vi "Append Paragraph.vi"(0 "PDF Report":refnum<class "PDF Report Class.lvclass">, 1 "Path":path, 2 "Text":string, 3 "Paragraph indentation":T3, 7 "Image to Add [ ]":T1 {"Scale" format="%#_g %"}, 11 "error in (no error)":errorcluster, 12 "Font":T7={"Name"="", "Size"=-1.0, "Color"=0, "Style"={"Bold"=FALSE, "Italic"=FALSE, "Underline"=FALSE, "Strikeout"=FALSE}, "Type"={"Type&direction"=enum."Select", "Embedded"=FALSE, "Encoding"=""}}, 14 "Paragraph properties":T4) -> (4 "PDF Report duplicate":refnum<class "PDF Report Class.lvclass">, 15 "error out":errorcluster)   [LabVIEW 2020, in "Exaprom PDF.lvlib"]
doc: "<B>Only ASCII or UTF-16 (no-bidi).</B>\n\nAppends text with a <B>line feed</B>, at the end, to the PDF report. This text can be <B>aligned</B> (CENTER, JUSTIFY, LEFT, RIGHT) and <B>indented</B>. \n\nIf <B>Font</B> and <B>Pararaph properties</B> are not specified then the <B>Default font</B> and <B>Default paragraph</B> will be use.\n\nThe data type you wire to the <B>Text</B> input determines the polymorphic instance to use.\n\n<B>FRANÇAIS</B>\nAjoute au rapport PDF du texte sous la forme d'un paragraphe terminé avec un \"<B>Line Feed</B>\". Ce texte peut être <B>aligné</B> (CENTER, JUSTIFY, LEFT, RIGHT) et avoir un <B>renfoncement</B> (gauche et droit) pour tout le paragraphe.\n\nSi la police de caractères <B>Font</B> et les propriétés <B>Pararaph properties</B> ne sont pas spécifiés alors la police par défaut <B>Default font</B> et <B>Default paragraph</B> seront utilisées.\n\nLe type de données que vous connectez au terminal <B>Text</B> détermine l'instance polymorphique utilisée.\n\nVersion 2.0\nDeveloped by Jean-Marc Simard\nCopyright © 2013, Exaprom Inc.\nAll rights reserved.\nLicense: BSD\n\nWith iTextSharp 4.1.6 (http://itextsharp.sourceforge.net)\nunder Mozilla Public License Version 1.1\n(http://www.mozilla.org/MPL/MPL-1.1.html)"
uses:
  <userlib>/labview-PDF-writer-master/Exaprom PDF.lvlib
  <userlib>/labview-PDF-writer-master/Controls/Font Controls/Font complete cluster.ctl
  <userlib>/labview-PDF-writer-master/Controls/Font Controls/Font size.ctl
  <userlib>/labview-PDF-writer-master/Controls/Font Controls/Font color.ctl
  <userlib>/labview-PDF-writer-master/Controls/Font Controls/Type and encoding.ctl
  <userlib>/labview-PDF-writer-master/Controls/Text Controls/Unicode/Type and run direction.ctl
  <userlib>/labview-PDF-writer-master/Controls/Initialization Controls/Defaut Paragraphe and Line Spacing.ctl
  <userlib>/labview-PDF-writer-master/Controls/Text Controls/Texte alignement.ctl
  <userlib>/labview-PDF-writer-master/Controls/Text Controls/Line spacing.ctl
  <userlib>/labview-PDF-writer-master/LV Class/PDF Report Class/PDF Report Class.lvclass
  <userlib>/labview-PDF-writer-master/Controls/Text Controls/Paragraph indentation.ctl
  <userlib>/labview-PDF-writer-master/Controls/General Controls/Image to Add [ ].ctl
  <userlib>/labview-PDF-writer-master/Controls/Image Controls/Image Scale.ctl
  <userlib>/labview-PDF-writer-master/Controls/Text Controls/Phrase or paragraph.ctl
  <userlib>/labview-PDF-writer-master/Controls/Text Controls/Unicode/Source rub direction.ctl
  C:/Program Files (x86)/National Instruments/LabVIEW 2020/user.lib/labview-PDF-writer-master/DLL/itextsharp.dll
  DLL/itextsharp.dll
  <userlib>/labview-PDF-writer-master/LV Class/Fonts Class/Font Class.lvclass
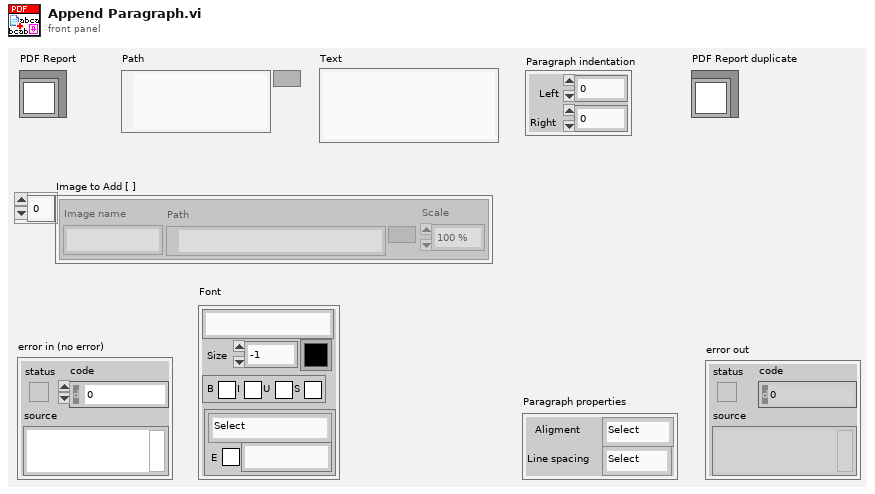
[diagram p1: front panel]
types:
  T1 = typedef "Exaprom PDF.lvlib/Image to Add [ ].ctl" = cluster{"Image name":string, "Path":path, "Scale":T2}[]
  T2 = typedef "Exaprom PDF.lvlib/Image Scale.ctl" = sgl
  T3 = typedef "Exaprom PDF.lvlib/Paragraph indentation.ctl" = cluster{"Left":sgl, "Right":sgl}
  T4 = typedef "Exaprom PDF.lvlib/Defaut Paragraphe and Line Spacing.ctl" = cluster{" Aligment":T5, "Line spacing":T6}
  T5 = typedef "Exaprom PDF.lvlib/Texte alignement.ctl" = enum16{"Select", "CENTER", "JUSTIFY", "LEFT", "RIGHT"}
  T6 = typedef "Exaprom PDF.lvlib/Line spacing.ctl" = enum16{"Select", "1.0", "1.5", "2.0"}
  T7 = typedef "Exaprom PDF.lvlib/Font complete cluster.ctl" = cluster{"Name":string, "Size":T8, "Color":T9, "Style":cluster{"Bold":bool, "Italic":bool, "Underline":bool, "Strikeout":bool}, "Type":T10}
  T8 = typedef "Exaprom PDF.lvlib/Font size.ctl" = sgl
  T9 = typedef "Exaprom PDF.lvlib/Font color.ctl" = u32
  T10 = typedef "Exaprom PDF.lvlib/Type and encoding.ctl" = cluster{"Type&direction":T11, "Embedded":bool, "Encoding":string}
  T11 = typedef "Exaprom PDF.lvlib/Type and run direction.ctl" = enum16{"Select", "ASCII", "UTF-16", "UTF-16 (default)", "UTF-16 (LTR)", "UTF-16 (RTL)"}
  T12 = typedef "Exaprom PDF.lvlib/Source rub direction.ctl" = enum16{"Chapter", "Paragraph", "Phrase", "pdfpcell"}
  T13 = typedef "Exaprom PDF.lvlib/Phrase or paragraph.ctl" = enum16{"Add to Phrase", "Add to Paragraph", "Create Phrase", "Create Paragraph"}
  T14 = typedef "Exaprom PDF.lvlib/Unit.ctl" = enum16{"inch", "mm"}
  T15 = typedef "Exaprom PDF.lvlib/Image to Add refnum [ ].ctl" = cluster{"Image name":string, "InstanceImage":refnum<k24>}[]
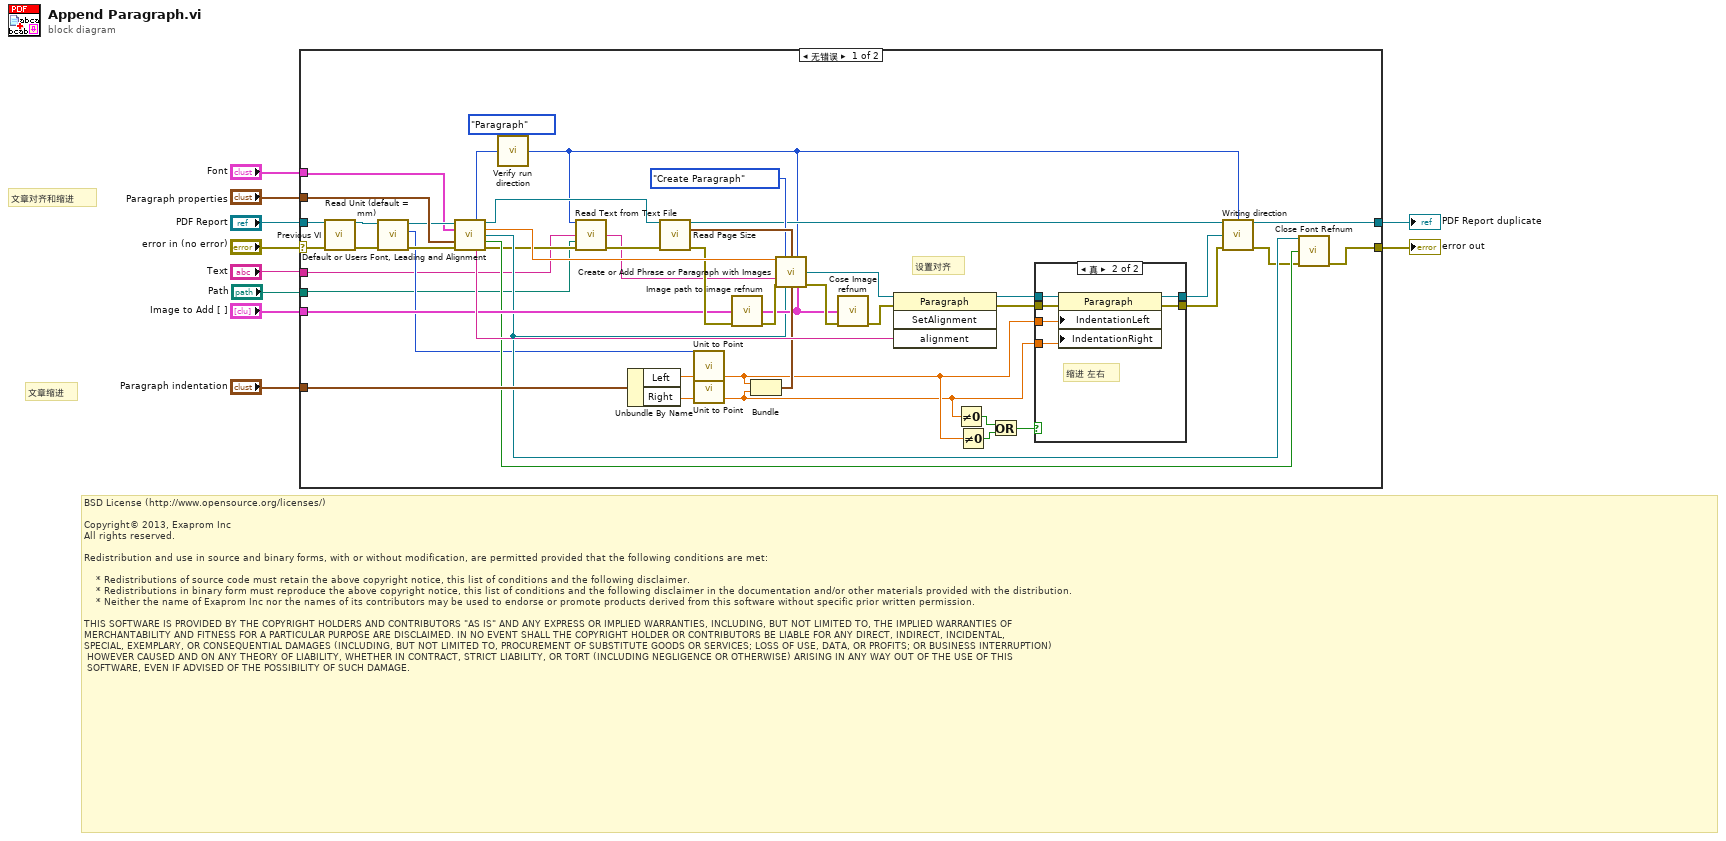
[diagram p0: block diagram]
diagram:
  # "文章对齐和缩进"
  # "文章缩进"
  # "BSD License (http://www.opensource.org/licenses/)\n\nCopyright© 2013, Exaprom Inc\nAll rights reserved.\n\nRedistribution and use in source and binary forms, with or without modification, are permitted provided that the following conditions are met:\n\n    * Redistributions of source code must retain the above copyright notice, this list of conditions and the following disclaimer.\n    * Redistributions in binary form must reproduce the above copyright notice, this list of conditions and the following disclaimer in the documentation and/or other materials provided with the distribution.\n    * Neither the name of Exaprom Inc nor the names of its contributors may be used to endorse or promote products derived from this software without specific prior written permission.\n\nTHIS SOFTWARE IS PROVIDED BY THE COPYRIGHT HOLDERS AND CONTRIBUTORS \"AS IS\" AND ANY EXPRESS OR IMPLIED WARRANTIES, INCLUDING, BUT NOT LIMITED TO, THE IMPLIED WARRANTIES OF \nMERCHANTABILITY AND FITNESS FOR A PARTICULAR PURPOSE ARE DISCLAIMED. IN NO EVENT SHALL THE COPYRIGHT HOLDER OR CONTRIBUTORS BE LIABLE FOR ANY DIRECT, INDIRECT, INCIDENTAL,\nSPECIAL, EXEMPLARY, OR CONSEQUENTIAL DAMAGES (INCLUDING, BUT NOT LIMITED TO, PROCUREMENT OF SUBSTITUTE GOODS OR SERVICES; LOSS OF USE, DATA, OR PROFITS; OR BUSINESS INTERRUPTION)\n HOWEVER CAUSED AND ON ANY THEORY OF LIABILITY, WHETHER IN CONTRACT, STRICT LIABILITY, OR TORT (INCLUDING NEGLIGENCE OR OTHERWISE) ARISING IN ANY WAY OUT OF THE USE OF THIS\n SOFTWARE, EVEN IF ADVISED OF THE POSSIBILITY OF SUCH DAMAGE."
  n1 = case shown="无错误" "error in (no error)" {
    selector: "error in (no error)" -> [w28 w68]
    tunnel: "Font" -> [w21 _]
    tunnel: "Text" -> [w15 _]
    tunnel: [w37 w68] -> w9
    tunnel: "PDF Report" -> [w47 w67]
    tunnel: "Paragraph properties" -> [w43 _]
    tunnel: [w26 w67] -> w5
    tunnel: "Paragraph indentation" -> [w55 _]
    tunnel: "Image to Add [ ]" -> [w39 _]
    tunnel: "Path" -> [w16 _]
    frame No Error {
      # "设置对齐"
      n2 = call <userlib>:"Previous VI.vi"("PDF Report IN"=w47, "error in (no error)"=w28) -> ("PDF Report OUT"=w20:refnum<class "PDF Report Class.lvclass">, "error out"=w13:errorcluster)  [unwired: 12 out]
      n3 = call-dynamic "Read Unit (default = mm).vi"("error in (no error)"=w13, "PDF Report Class in"=w20) -> ("error out"=w34:errorcluster, "Unit (default = mm)"=w32:T14, "PDF Report Class out"=w33:refnum<class "PDF Report Class.lvclass">)  [unwired: 7 in]
      n4 = call <userlib>:"Default or Users Font, Leading and Alignment.vi"("PDF Report"=w33, "Font"=w21, "Paragraphe cluster"=w43, "error in (no error)"=w34) -> ("Type and run direction"=w17:T11, "PDF Report duplicate"=w40:refnum<class "PDF Report Class.lvclass">, "Leading"=w49:T8, "Font Ref"=w35:refnum<k24>, "Close Font Ref"=w36:bool, "Aligment"=w57:string, "error out"=w19:errorcluster)  [unwired: 5 out]
      n5 = call <userlib>:"Verify run direction.vi"("Source"=Source_rub_direction."Paragraph", "Type&direction IN"=w17) -> ("Type&direction OUT"=w12:T11)  [unwired: 2 in]
      n6 = call <userlib>:"Read Text from Text File.vi"("Text and direction IN"=w12, "Text IN"=w15, "Path"=w16, "error in (no error)"=w19) -> ("Text OUT"=w14:string, "error out"=w18:errorcluster)  [unwired: 9 in, 1 out]
      n7 = Unbundle By Name(w55) -> ("Left"=w51:sgl, "Right"=w50:sgl)
      n8 = call <userlib>:"Read Page Size.vi"("PDF Report"=w40, "error in (no error)"=w18) -> ("PDF Report duplicate"=w25:refnum<class "PDF Report Class.lvclass">, "Text zone (points)"=w42:cluster{"widht":sgl, "height":sgl}, "error out"=w41:errorcluster)  [unwired: 11 out]
      n9 = call <userlib>:"Unit to Point.vi"("X unit"=w51, "Unit (default = mm)"=w32) -> ("X point"=w30:sgl)  [unwired: 7 out]
      n10 = call <userlib>:"Unit to Point.vi"("X unit"=w50, "Unit (default = mm)"=w32) -> ("X point"=w29:sgl)  [unwired: 7 out]
      n11 = call <userlib>:"Image path to image refnum.vi"("Image to Add [ ]"=w39, "error in (no error)"=w41) -> ("Image to Add refnum [ ]"=w38:T15, "error out"=w58:errorcluster)  [unwired: 2 in, 10 out]
      n12 = Bundle("X point"=w30, "X point"=w29) -> (w46:cluster{" X point":sgl, " X point":sgl})  [unwired: 1 out]
      n13 = call <userlib>:"Create or Add Phrase or Paragraph with Images.vi"("Leading"=w49, "Phrase or paragraph"=Phrase_or_paragraph."Create Paragraph", "Text zone (points)"=w42, "Character type"=w12, "Text"=w14, "error in (no error)"=w58, "Font refnum"=w35, "Paragraph indentation (points)"=w46, "Image to Add refnum [ ]"=w38) -> ("Paragraph refnum OUT"=w48:refnum<k24>, "error out"=w45:errorcluster)  [unwired: 2 in, 3 out]
      n14 = call <userlib>:"Cose Image refnum.vi"("Image to Add refnum [ ]"=w38, "error in (no error)"=w45) -> ("error out"=w44:errorcluster)  [unwired: 13 out]
      n15 = invoke class="Paragraph" method="SetAlignment"(reference=w48, error in=w44, "alignment"=w57) -> (reference out=w24:refnum<k24>, error out=w56:errorcluster)  [unwired: 1 in, 2 out]
      n16 = Not Equal To 0?(x=w29) -> (x != 0?=w53:bool)
      n17 = Not Equal To 0?(x=w30) -> (x != 0?=w52:bool)
      n18 = Or(x=w53, y=w52) -> (x .or. y?=w54:bool)
      n19 = case shown="真" w54 {
        tunnel: w24 -> [w60 w66]
        tunnel: w56 -> [w59 w65]
        tunnel: [w59 w64] -> w23
        tunnel: [w60 w63] -> w22
        tunnel: w30 -> [_ w62]
        tunnel: w29 -> [_ w61]
        frame False {
        }
        frame True {
          # "缩进 左右"
          n20 = property class="Paragraph"(reference=w66, error in=w65, "IndentationLeft"=w62, "IndentationRight"=w61) -> (reference out=w63:refnum<k24>, error out=w64:errorcluster)
        }
      }
      n21 = call <userlib>:"Writing direction.vi"("PDF Report IN"=w25, "Text type"=w12, "Paragraph refnum"=w22, "error in (no error)"=w23) -> ("PDF Report OUT"=w26:refnum<class "PDF Report Class.lvclass">, "error out"=w27:errorcluster)  [unwired: 10 in]
      n22 = call <userlib>:"Close Font Refnum.vi"("Font Refnum"=w35, "Close ?"=w36, "error in (no error)"=w27) -> ("error out"=w37:errorcluster)  [unwired: 12 in]
    }
    frame Error {
    }
  }
  "error out" <- w9
  "PDF Report duplicate" <- w5
